vi "spindisk_unit_controller.vi"() -> ()   [LabVIEW 2016]
uses:
  <vilib>/Utility/error.llb/DialogType.ctl
  <vilib>/DAQmx/read.llb/DAQmx Read (Analog 1D DBL NChan 1Samp).vi
  <vilib>/DAQmx/miscellaneous.llb/DAQmx Fill In Error Info.vi
panel:
  in  "quit":bool
  in  "Spinning disk tab":enum32{"BD-CRVII", "ASI & Config File Info"}(tab)
  out "Ext Control Status":bool
  in  "Ext. analog control switch":bool
  in  "Analog control device":tag
  in  "Emission Filter":u16(ring) items=["Unknown Filter 1", "Unknown Filter 2", "Unknown Filter 3", "Unknown Filter 4", "Unknown Filter 5", "Unknown Filter 6", "Unknown Filter 7", "Unknown Filter 8"]
  in  "Dichroic Mirror":u16(ring) items=["Unknown Filter 1", "Unknown Filter 2", "Unknown Filter 3", "Unknown Filter 4", "Unknown Filter 5"]
  in  "Excitation Filter":u16(ring) items=["Unknown Filter 1", "Unknown Filter 2", "Unknown Filter 3", "Unknown Filter 4", "Unknown Filter 5", "Unknown Filter 6", "Unknown Filter 7", "Unknown Filter 8"]
  out "COM status":bool
  in  "Port Name":refnum<visa-resource-name>
  in  "Disk position":bool
  in  "Disk spinning":bool
  in  "Shutter":bool
  in  "init":bool
  in  "Ext. TTL Shutter\n Control":bool
  in  "ext. control update time (ms)":i32=50
  in  "serial response delay (ms)":u32
  in  "ext. cmd update delay (ms)":u32=500 max=1000
  out "cmd string":string
  out "Firmware Version":string
  out "query response":string
  out "ext. sig.\ncommitted":bool
  out "analog inputs":dbl[](array[numeric]) caption="analog \ninputs" format="%#1.3f"
  out "ASI REEPONSE":string
  out "ASI CMD":string
  in  "ASI Stage Port":refnum<visa-resource-name>
  in  "Set Backlash Values":bool
  in  "X backlash (um)":dbl min=0.0 max=200.0 step=0.5
  in  "Y backlash (um)":dbl min=0.0 max=200.0 step=0.5
  in  "Z backlash (um)":dbl=-40.0 min=-200.0 max=200.0 step=0.5
  out "Configuration file":string
  out "error out":errorcluster
  # "Programmed by Quan Qing\nQingLAB@ASU\nhttp://qinglab.physics.asu.edu\nquan.qing@asu.edu"
  # "ExFilter"
  # "EmFilter"
  # "DiMirror"
  # "DiskPos"
  # "DiskSpin"
  # "ASI backslash setting"
  # "Config. file information"
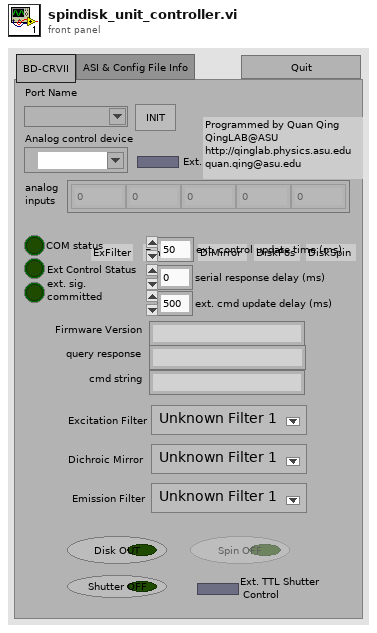
[diagram p1: front panel]
types:
  T1 = enum8{"Enabled", "Disabled", "Disabled and Grayed Out"}
  T2 = typedef "DialogType.ctl" = u16
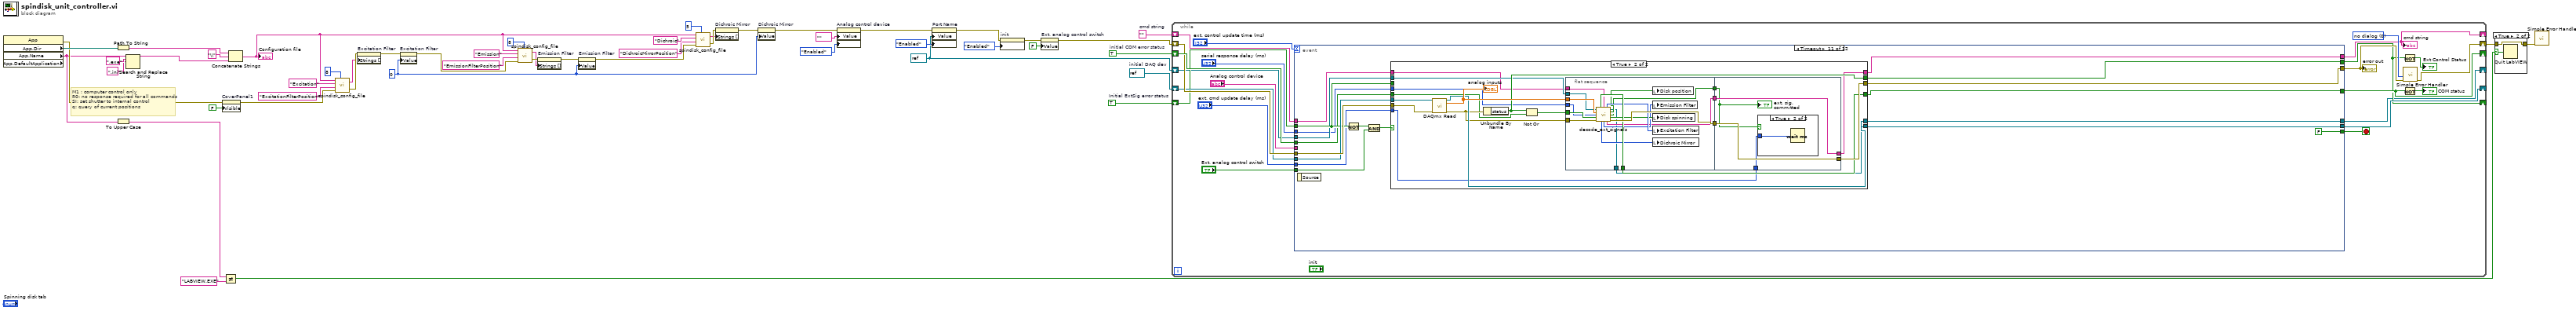
[diagram p0: block diagram]
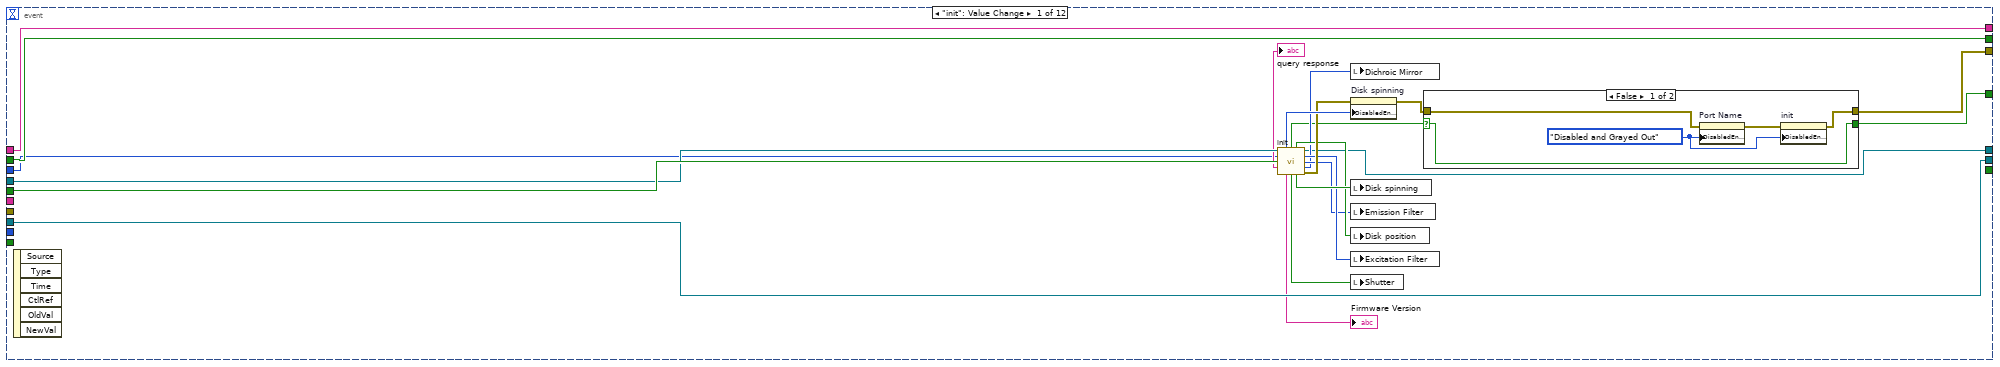
[diagram p3: hidden frame]
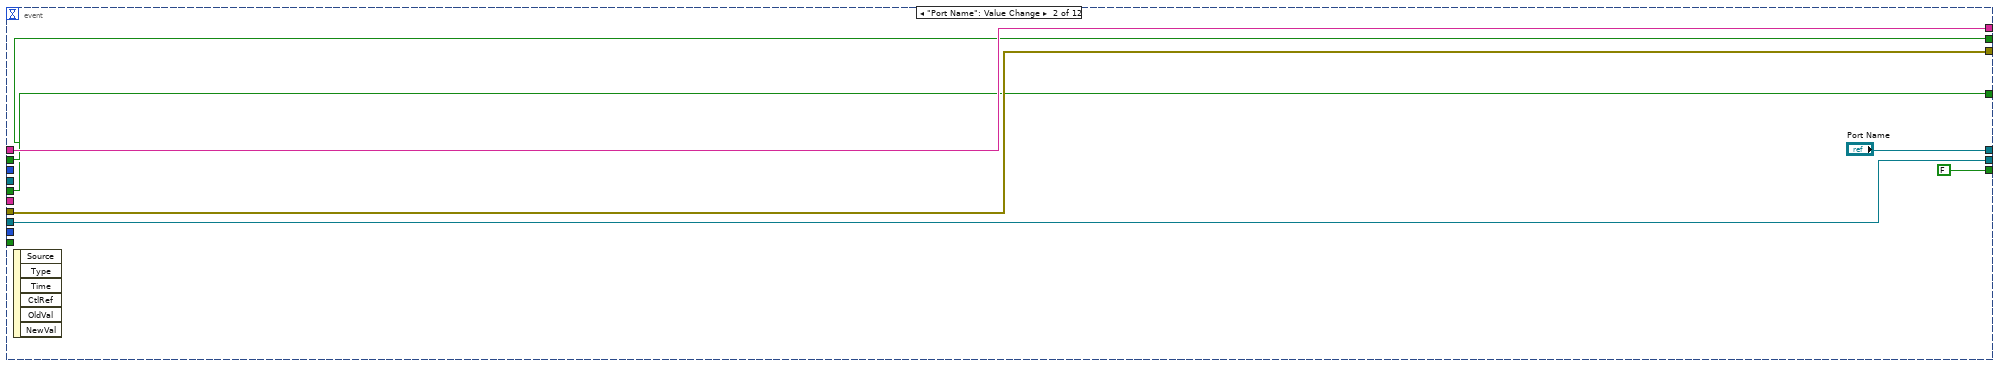
[diagram p5: hidden frame]
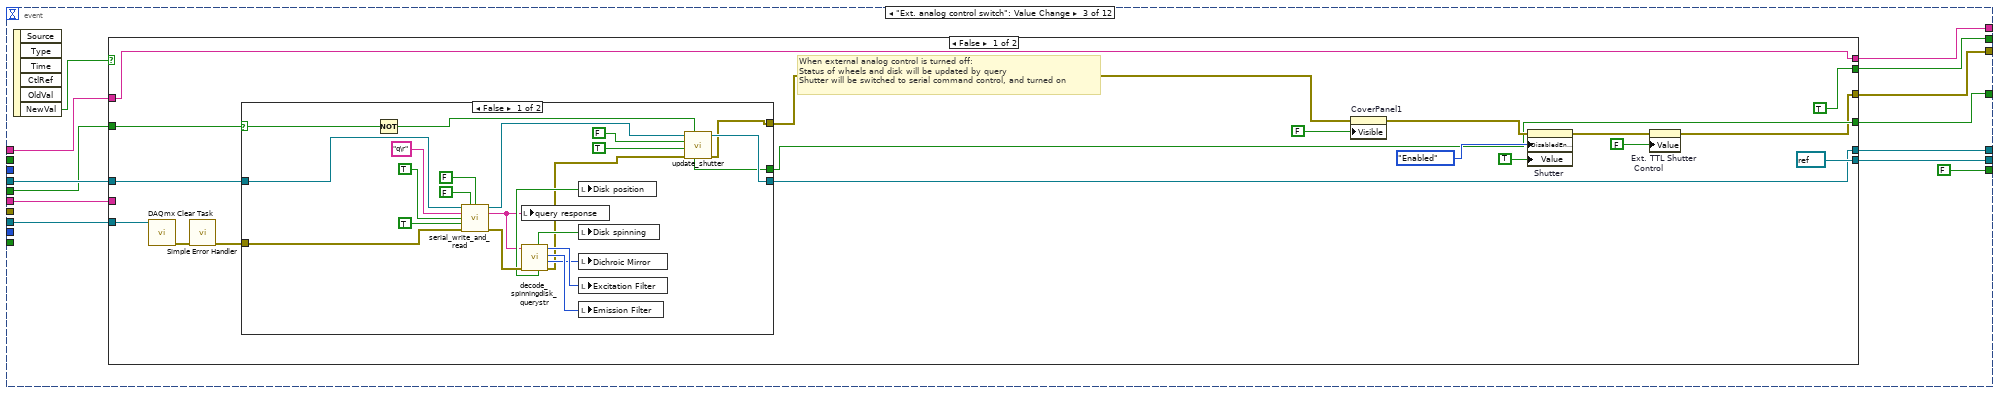
[diagram p6: hidden frame]
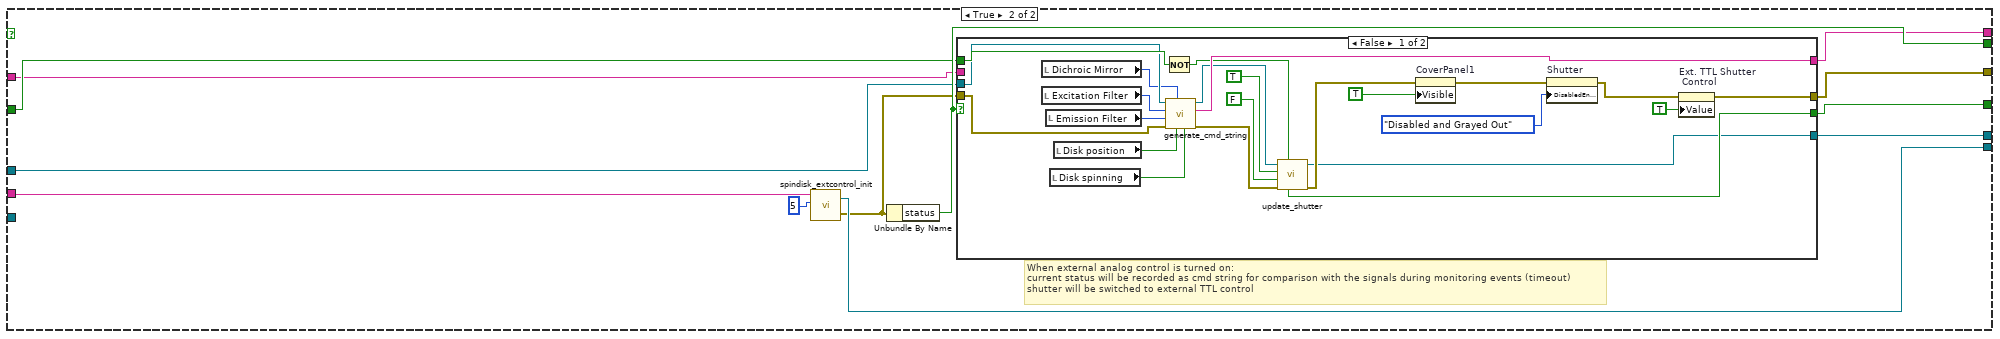
[diagram p8: hidden frame]
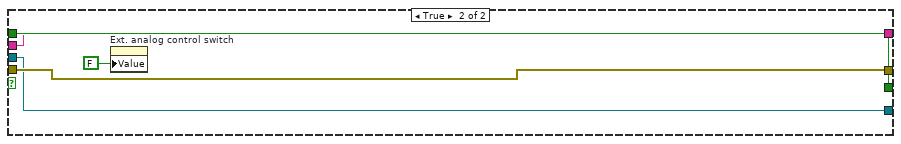
[diagram p9: hidden frame]
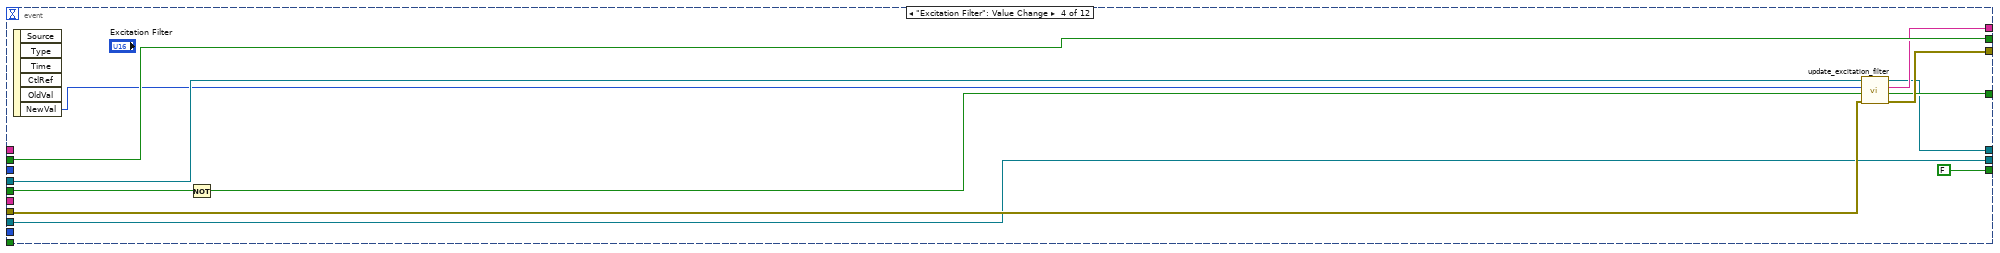
[diagram p10: hidden frame]
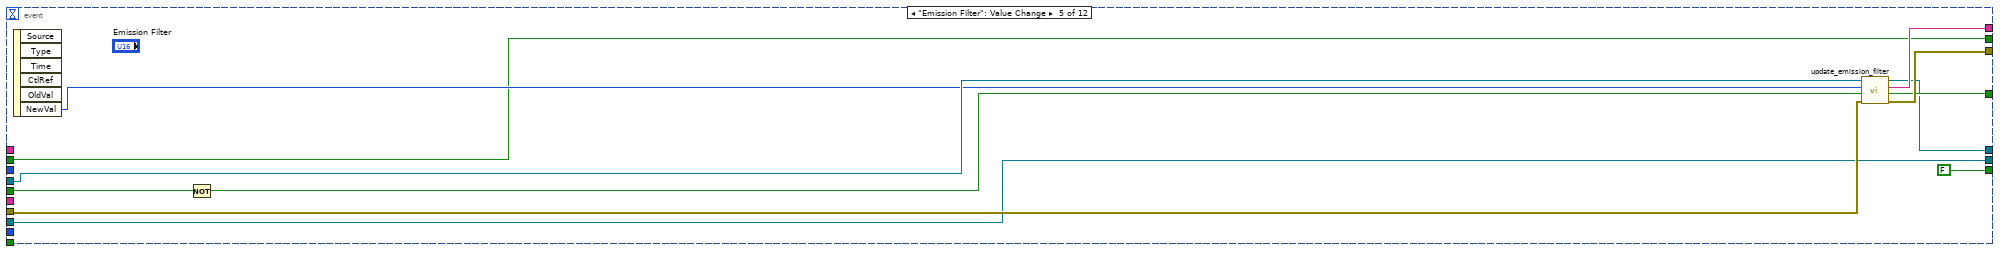
[diagram p11: hidden frame]
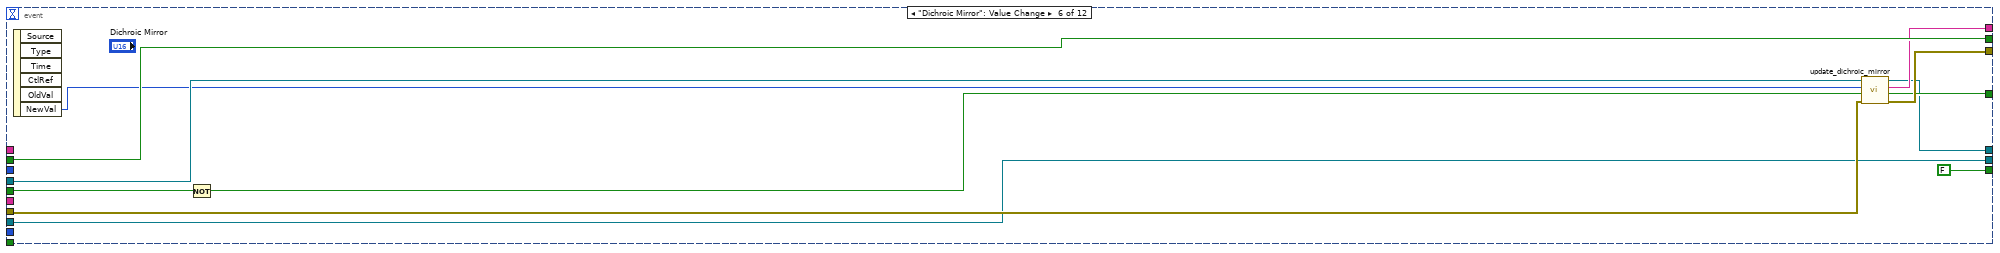
[diagram p12: hidden frame]
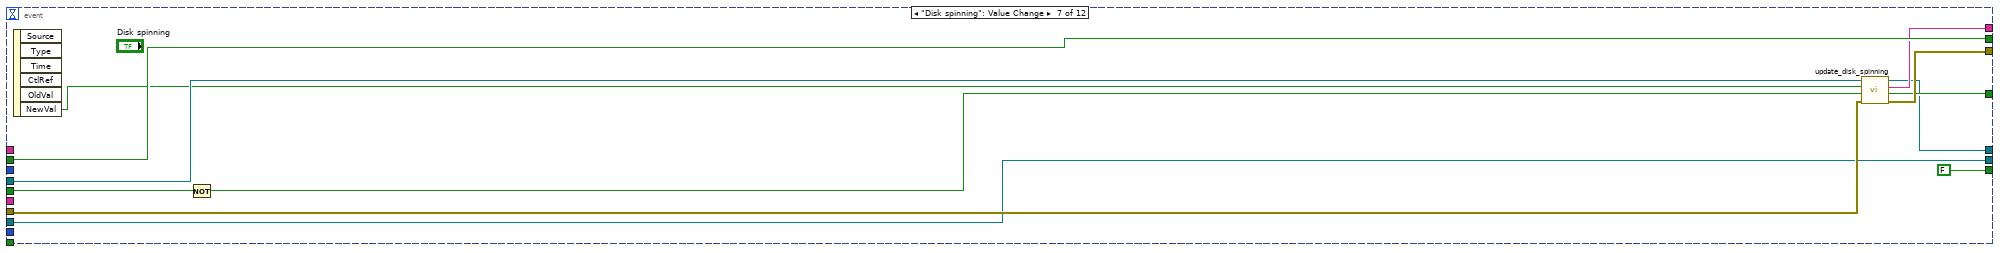
[diagram p13: hidden frame]
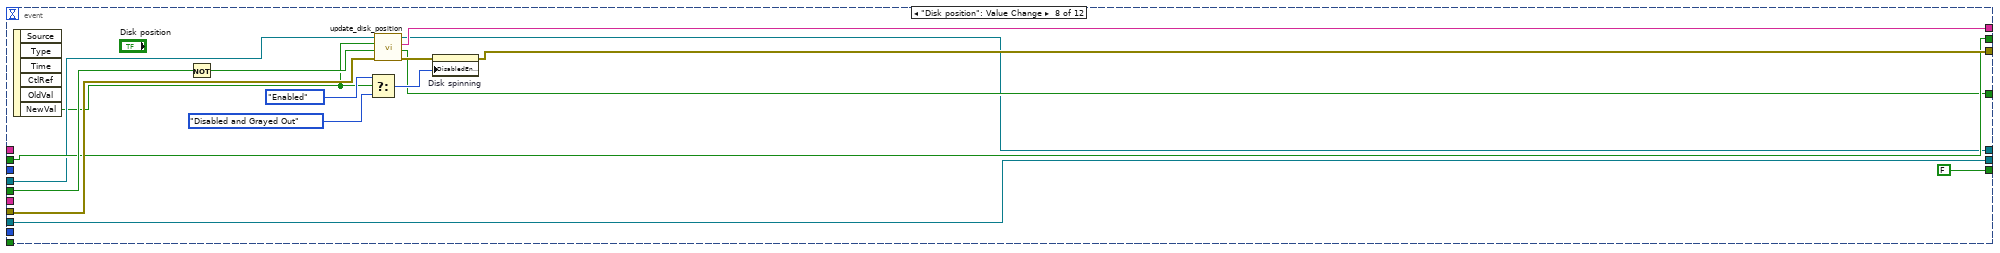
[diagram p14: hidden frame]
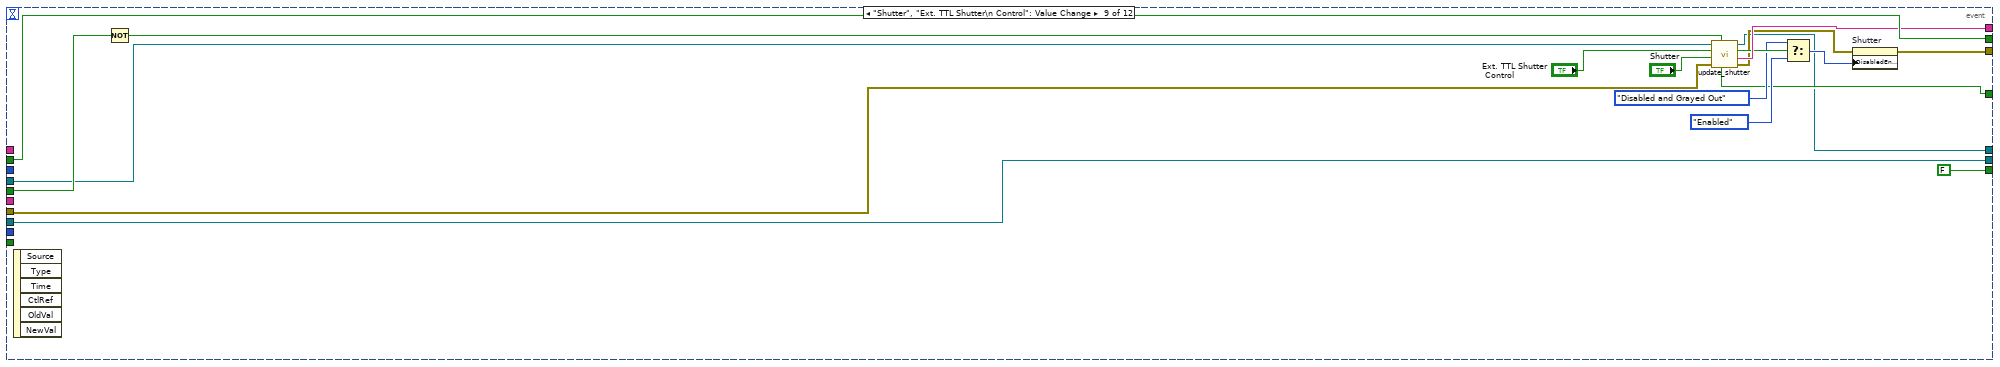
[diagram p15: hidden frame]
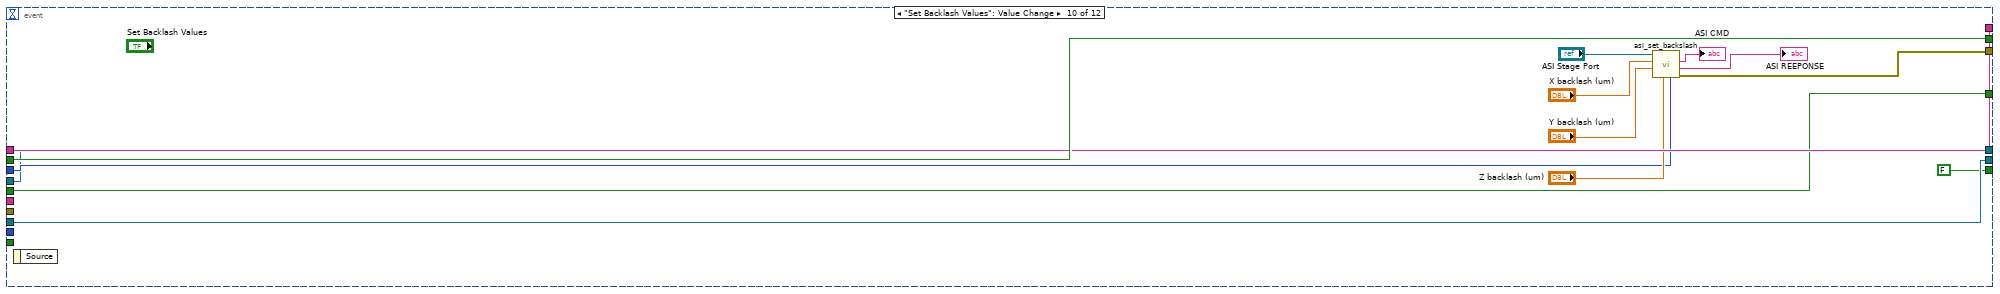
[diagram p16: hidden frame]
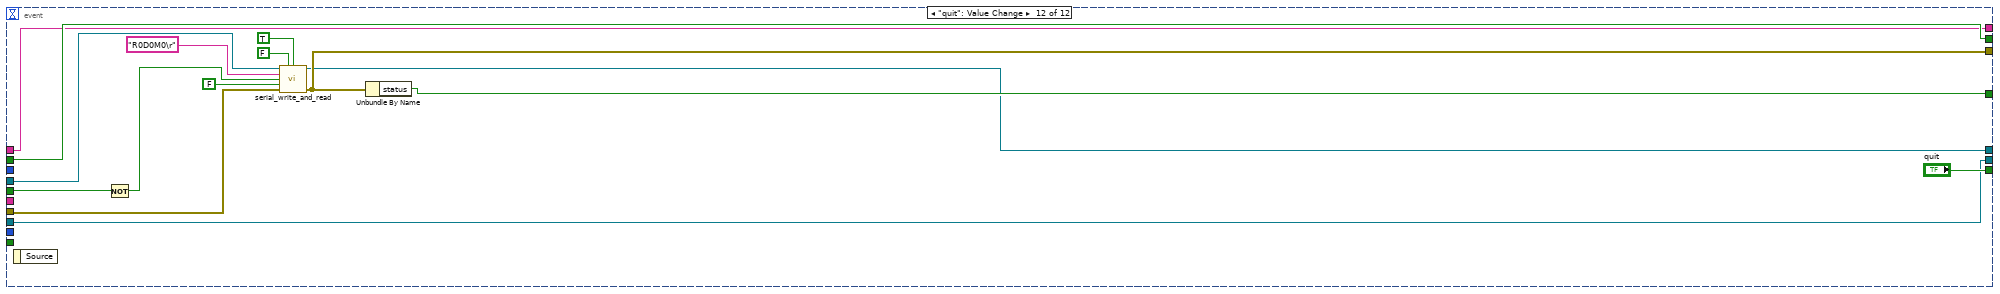
[diagram p19: hidden frame]
diagram:
  w3 = refnum<visa-resource-name> refnum ("Port Name")
  w16 = ""  # cmd string
  w19 = refnum<k21> refnum  # initial DAQ dev
  w18 = TRUE  # Initial ExtSig error status
  w26 = u16 0
  w36 = TRUE  # initial COM error status
  # "M1 : computer control only\nR0: no response required for all commands\nSI: set shutter to internal control\nq: query of current positions"
  n1 = property class="App" props=["App.Dir", "App.Name", "App.DefaultApplication"]() -> (error out=w15:errorcluster, "App.Dir"=w50:path, "App.Name"=w1:string)  [unwired: 2 in, 2 out]
  n2 = Path To String(path=w50) -> (string=w49:string)
  n3 = To Upper Case(1:w1) -> (0:w21:string)
  n4 = Search and Replace String(input string=w1, search string=".exe", replace string=".ini" ("replace string (\"\")")) -> (result string=w47:string)  [unwired: 5 in, 3 out]
  n5 = property on="CoverPanel1" class="SubPnl"(error in=w15, "Visible"=FALSE) -> (error out=w2:errorcluster)  [unwired: 1 in, 1 out]
  n6 = Not Equal?(x=w21, y="LABVIEW.EXE") -> (x != y?=w17:bool)
  n7 = Concatenate Strings(w49, "\\" ("string"), w47) -> (w42:string)
  "Configuration file" <- w42
  n8 = call "spindisk_config_file.vi"("config file path name"=w42, "section"="Excitation", "common_keyname"="ExcitationFilterPosition", "error in (no error)"=w2, "Positions"=8) -> ("filter list"=w25:string[], "error out"=w33:errorcluster)
  n9 = property on="Excitation Filter" class="Ring (strict)"(error in=w33, "Strings []"=w25) -> (error out=w34:errorcluster)  [unwired: 1 in, 1 out]
  n10 = property on="Excitation Filter" class="Ring (strict)"(error in=w34, "Value"=w26) -> (error out=w32:errorcluster)  [unwired: 1 in, 1 out]
  n11 = call "spindisk_config_file.vi"("config file path name"=w42, "section"="Emission", "common_keyname"="EmissionFilterPosition", "error in (no error)"=w32, "Positions"=8) -> ("filter list"=w24:string[], "error out"=w31:errorcluster)
  n12 = property on="Emission Filter" class="Ring (strict)"(error in=w31, "Strings []"=w24) -> (error out=w30:errorcluster)  [unwired: 1 in, 1 out]
  n13 = property on="Emission Filter" class="Ring (strict)"(error in=w30, "Value"=w26) -> (error out=w29:errorcluster)  [unwired: 1 in, 1 out]
  n14 = call "spindisk_config_file.vi"("config file path name"=w42, "section"="Dichroic", "common_keyname"="DichroicMirrorPosition", "error in (no error)"=w29, "Positions"=5) -> ("filter list"=w23:string[], "error out"=w28:errorcluster)
  n15 = property on="Dichroic Mirror" class="Ring (strict)"(error in=w28, "Strings []"=w23) -> (error out=w27:errorcluster)  [unwired: 1 in, 1 out]
  n16 = property on="Dichroic Mirror" class="Ring (strict)"(error in=w27, "Value"=w26) -> (error out=w7:errorcluster)  [unwired: 1 in, 1 out]
  n17 = property on="Analog control device" class="DAQmxName"(error in=w7, "Value"=tag "" ("Ext I/O device"), "DisabledEnum"=T1."Enabled" ("Disabled")) -> (error out=w6:errorcluster)  [unwired: 1 in, 1 out]
  n18 = property on="Port Name" class="VISAName"(error in=w6, "Value"=w3, "DisabledEnum"=T1."Enabled" ("Disabled")) -> (error out=w5:errorcluster)  [unwired: 1 in, 1 out]
  n19 = property on="init" class="Bool"(error in=w5, "DisabledEnum"=T1."Enabled" ("Disabled")) -> (error out=w4:errorcluster)  [unwired: 1 in, 1 out]
  n20 = property on="Ext. analog control switch" class="Bool (strict)"(error in=w4, "Value"=FALSE ("Ext. control enabled")) -> (error out=w13:errorcluster)  [unwired: 1 in, 1 out]
  n21 = while {
    shift-right: [w71] -> _
    shift-left: w36 -> [w73]
    shift-right: [w64] -> w22
    shift-left: w13 -> [w72]
    shift-right: [w68] -> _
    shift-left: w19 -> [w69]
    shift-right: [w62] -> _
    shift-left: w18 -> [w66]
    shift-right: [w59] -> _
    shift-left: w16 -> [w58]
    shift-right: [w53] -> _
    shift-left: w3 -> [w54]
    stop <- w74 stop-if-true
    w63 = T2 0 items=["no dialog", "OK message", "continue or stop message", "OK message + warnings", "continue/stop + warnings"] ("type of dialog (OK msg:1)")
    n22 = event shown="[10] Timeout" {
      selector: _ -> [_ _ _ _ _ _ _ _ _ _ _ _]
      dyn-events: _ -> [_ _ _ _ _ _ _ _ _ _ _ _]
      timeout: "ext. control update time (ms)" -> [_ _ _ _ _ _ _ _ _ _ _ _]
      tunnel: [_ FALSE ("quit") FALSE ("quit") FALSE ("quit") FALSE ("quit") FALSE ("quit") FALSE ("quit") FALSE ("quit") FALSE ("quit") FALSE ("quit") FALSE ("quit") "quit"] -> w74
      tunnel: [w78 w103 w114 w210 w222 w234 w246 w258 w275 w290 w312 w372] -> w71
      tunnel: w73 -> [w95 w103 w115 w214 w228 w240 w251 w268 w280 w290 w313 w375]
      tunnel: [w77 w108 w120 w218 w230 w242 w254 w269 w288 w302 w319 w373] -> w65
      tunnel: w72 -> [_ w108 _ w217 w229 w239 w252 w270 w287 _ w320 w381]
      tunnel: w69 -> [w94 w106 w122 w209 w220 w231 w245 w256 w272 w301 w318 w367]
      tunnel: [w94 w106 w121 w209 w220 w231 w245 w256 w272 w301 w317 w367] -> w68
      tunnel: [w91 w104 w119 w216 w223 w241 w253 w267 w286 w300 w311 w380] -> w62
      tunnel: w66 -> [w91 w104 _ w216 w223 w241 w253 w267 w286 w300 w314 w380]
      tunnel: w54 -> [w90 _ w116 w212 w225 w236 w248 w260 w278 w289 w310 w369]
      tunnel: "Analog control device" -> [_ _ w118 _ _ _ _ _ _ _ _ _]
      tunnel: "Ext. analog control switch" -> [_ _ _ _ _ _ _ _ _ _ w309 _]
      tunnel: [w81 w107 w112 w215 w227 w238 w250 w266 w285 w297 w308 w370] -> w59
      tunnel: w58 -> [w81 w107 w113 _ _ _ _ _ _ w297 w307 w370]
      tunnel: "ext. cmd update delay (ms)" -> [_ _ _ _ _ _ _ _ _ _ w306 _]
      tunnel: "serial response delay (ms)" -> [w76 _ _ _ _ _ _ _ _ w292 w305 _]
      tunnel: [w75 "Port Name" w111 w208 w221 w232 w244 w257 w273 w289 w303 w368] -> w53
      event "init": Value Change {
        n23 = event-data() -> ()  [unwired: 1 in, 6 out]
        n24 = call "init.vi"("Port Name"=w90, "COM response delay"=w76, "current error status"=w95) -> ("disk spinning disable state"=w93:T1, "new error status"=w80:bool, "Disk position"=w87:bool, "VISA resource name out"=w75:refnum<visa-resource-name>, "Excitation Filter"=w86:u16, "Emission Filter"=w85:u16, "query response"=→"query response":string, "Dichroic Mirror"=w84:u16, "Firmware Version"=→"Firmware Version":string, "Shutter"=w89:bool, "Disk spinning"=w88:bool, "error out"=w92:errorcluster)  [unwired: 1 in]
        n25 = local write "Dichroic Mirror"(w84) -> ()
        n26 = property on="Disk spinning" class="Bool (strict)"(error in=w92, "DisabledEnum"=w93) -> (error out=w79:errorcluster)  [unwired: 1 in, 1 out]
        n27 = local write "Disk spinning"(w88) -> ()
        n28 = local write "Emission Filter"(w85) -> ()
        n29 = local write "Disk position"(w87) -> ()
        n30 = local write "Excitation Filter"(w86) -> ()
        n31 = local write "Shutter"(w89) -> ()
        n32 = case shown="False" w80 {
          selector: w80 -> [w100 w102]
          tunnel: w79 -> [w99 w101]
          tunnel: [w100 w102] -> w78
          tunnel: [w97 w101] -> w77
          frame False {
            w96 = T1."Disabled and Grayed Out" ("Disabled")
            n33 = property on="Port Name" class="VISAName"(error in=w99, "DisabledEnum"=w96) -> (error out=w98:errorcluster)  [unwired: 1 in, 1 out]
            n34 = property on="init" class="Bool"(error in=w98, "DisabledEnum"=w96) -> (error out=w97:errorcluster)  [unwired: 1 in, 1 out]
          }
          frame True {
          }
        }
      }
      event "Port Name": Value Change {
        n35 = event-data() -> ()  [unwired: 1 in, 6 out]
      }
      event "Ext. analog control switch": Value Change {
        n36 = event-data() -> ("NewVal"=w117:bool)  [unwired: 1 in, 5 out]
        n37 = case shown="False" w117 {
          tunnel: w118 -> [_ w178]
          tunnel: [w125 w173] -> w120
          tunnel: [refnum<k21> refnum ("task out") w176] -> w121
          tunnel: w122 -> [w140 _]
          tunnel: [TRUE ("status") w175] -> w119
          tunnel: w116 -> [w127 w172]
          tunnel: w115 -> [w124 w171]
          tunnel: [w126 w170] -> w114
          tunnel: w113 -> [w130 w169]
          tunnel: [w130 w168] -> w112
          tunnel: [w123 w167] -> w111
          frame False {
            # "When external analog control is turned off:\nStatus of wheels and disk will be updated by query\nShutter will be switched to serial command control, and turned on"
            n38 = call <vilib>:"DAQmx Clear Task.vi"("task in"=w140) -> ("error out"=w139:errorcluster)  [unwired: 14 in]
            n39 = call <vilib>:"Simple Error Handler.vi"("error in (no error)"=w139) -> ("error out"=w129:errorcluster)  [unwired: 4 in, 4 out]
            n40 = case shown="False" w124 {
              selector: w124 -> [w146 w164]
              tunnel: w129 -> [w157 w165]
              tunnel: [w143 w165] -> w128
              tunnel: w127 -> [w156 w166]
              tunnel: [w147 w166] -> w123
              tunnel: [w145 w164] -> w126
              frame False {
                n41 = Not(x=w146) -> (.not. x?=w142:bool)
                n42 = call "serial_write_and_read.vi"("port name in"=w156, "reconnect?"=FALSE, "disconnect?"=FALSE, "write buffer"="q\r", "do writing?"=TRUE, "expecting response?"=TRUE, "error in"=w157) -> ("port name out"=w148:refnum<visa-resource-name>, "read buffer"=w141:string, "error out"=w159:errorcluster)  [unwired: 6 in]
                n43 = local write "query response"(w141) -> ()
                n44 = call "decode_spinningdisk_querystr.vi"("input string"=w141, "error in"=w159) -> ("disk spinning"=w151:bool, "disk position"=w152:bool, "excitation filter"=w154:u16, "emission filter"=w155:u16, "dichroic mirror"=w153:u16, "error out"=w144:errorcluster)  [unwired: 2 in, 1 out]
                n45 = local write "Disk position"(w152) -> ()
                n46 = local write "Disk spinning"(w151) -> ()
                n47 = local write "Dichroic Mirror"(w153) -> ()
                n48 = local write "Excitation Filter"(w154) -> ()
                n49 = local write "Emission Filter"(w155) -> ()
                n50 = call "update_shutter.vi"("commit?"=w142, "error in"=w144, "Shutter"=TRUE, "TTL external control?"=FALSE, "port in"=w148) -> ("error out"=w143:errorcluster, "port out"=w147:refnum<visa-resource-name>, "update COM error status"=w145:bool)  [unwired: 2 out]
              }
              frame True {
              }
            }
            n51 = property on="CoverPanel1" class="SubPnl"(error in=w128, "Visible"=FALSE) -> (error out=w132:errorcluster)  [unwired: 1 in, 1 out]
            n52 = property on="Shutter" class="Bool (strict)"(error in=w132, "DisabledEnum"=T1."Enabled" ("Disabled"), "Value"=TRUE ("Shutter")) -> (error out=w136:errorcluster)  [unwired: 1 in, 1 out]
            n53 = property on="Ext. TTL Shutter\n Control" class="Bool (strict)"(error in=w136, "Value"=FALSE ("TTL Shutter Control")) -> (error out=w125:errorcluster)  [unwired: 1 in, 1 out]
          }
          frame True {
            # "When external analog control is turned on:\ncurrent status will be recorded as cmd string for comparison with the signals during monitoring events (timeout)\nshutter will be switched to external TTL control"
            n54 = call "spindisk_extcontrol_init.vi"("Choose Device"=w178, "Analog input number"=5) -> ("task out"=w176:refnum<k21>, "error out"=w174:errorcluster)  [unwired: 3 in]
            n55 = Unbundle By Name(w174) -> ("status"=w175:bool)
            n56 = case shown="False" w175 {
              tunnel: w174 -> [w195 w204]
              tunnel: [w187 w204] -> w173
              tunnel: w172 -> [w194 w202]
              tunnel: w171 -> [w199 w206]
              tunnel: [w181 w206] -> w170
              tunnel: w169 -> [_ w203]
              tunnel: [w193 w203] -> w168
              tunnel: [w179 w202] -> w167
              frame False {
                n57 = local read "Dichroic Mirror"() -> (w192:u16)
                n58 = local read "Excitation Filter"() -> (w190:u16)
                n59 = local read "Emission Filter"() -> (w189:u16)
                n60 = local read "Disk spinning"() -> (w191:bool)
                n61 = local read "Disk position"() -> (w188:bool)
                n62 = Not(x=w199) -> (.not. x?=w180:bool)
                n63 = call "generate_cmd_string.vi"("disk spinning"=w191, "disk position"=w188, "dichroic mirror"=w192, "error in (no error)"=w195, "emission filter"=w189, "excitation filter"=w190, "port in"=w194) -> ("error out"=w183:errorcluster, "cmd string"=w193:string, "port out"=w184:refnum<visa-resource-name>)  [unwired: 2 in]
                n64 = call "update_shutter.vi"("commit?"=w180, "error in"=w183, "Shutter"=FALSE, "TTL external control?"=TRUE, "port in"=w184) -> ("error out"=w182:errorcluster, "port out"=w179:refnum<visa-resource-name>, "update COM error status"=w181:bool)  [unwired: 2 out]
                n65 = property on="CoverPanel1" class="SubPnl"(error in=w182, "Visible"=TRUE) -> (error out=w197:errorcluster)  [unwired: 1 in, 1 out]
                n66 = property on="Shutter" class="Bool (strict)"(error in=w197, "DisabledEnum"=T1."Disabled and Grayed Out" ("Disabled")) -> (error out=w201:errorcluster)  [unwired: 1 in, 1 out]
                n67 = property on="Ext. TTL Shutter\n Control" class="Bool (strict)"(error in=w201, "Value"=TRUE ("TTL Shutter Control")) -> (error out=w187:errorcluster)  [unwired: 1 in, 1 out]
              }
              frame True {
                n68 = property on="Ext. analog control switch" class="Bool (strict)"("Value"=FALSE ("Ext. control enabled")) -> ()  [unwired: 2 in, 2 out]
              }
            }
          }
        }
      }
      event "Excitation Filter": Value Change {
        n69 = event-data() -> ("NewVal"=w211:u16)  [unwired: 1 in, 5 out]
        n70 = Not(x=w214) -> (.not. x?=w213:bool)
        n71 = call "update_excitation_filter.vi"("error in (no error)"=w217, "commit?"=w213, "excitation filter #"=w211, "VISA resource name"=w212) -> ("error out"=w218:errorcluster, "update COM error status"=w210:bool, "cmd string"=w215:string, "VISA resource name out"=w208:refnum<visa-resource-name>)
      }
      event "Emission Filter": Value Change {
        n72 = event-data() -> ("NewVal"=w224:u16)  [unwired: 1 in, 5 out]
        n73 = Not(x=w228) -> (.not. x?=w226:bool)
        n74 = call "update_emission_filter.vi"("error in (no error)"=w229, "commit?"=w226, "emission filter #"=w224, "VISA resource name"=w225) -> ("error out"=w230:errorcluster, "update COM error status"=w222:bool, "cmd string"=w227:string, "VISA resource name out"=w221:refnum<visa-resource-name>)
      }
      event "Dichroic Mirror": Value Change {
        n75 = event-data() -> ("NewVal"=w235:u16)  [unwired: 1 in, 5 out]
        n76 = Not(x=w240) -> (.not. x?=w237:bool)
        n77 = call "update_dichroic_mirror.vi"("error in (no error)"=w239, "commit?"=w237, "dichroic mirror #"=w235, "VISA resource name"=w236) -> ("error out"=w242:errorcluster, "update COM error status"=w234:bool, "cmd string"=w238:string, "VISA resource name out"=w232:refnum<visa-resource-name>)
      }
      event "Disk spinning": Value Change {
        n78 = event-data() -> ("NewVal"=w247:bool)  [unwired: 1 in, 5 out]
        n79 = Not(x=w251) -> (.not. x?=w249:bool)
        n80 = call "update_disk_spinning.vi"("error in (no error)"=w252, "commit?"=w249, "disk spinning"=w247, "VISA resource name"=w248) -> ("error out"=w254:errorcluster, "update COM error status"=w246:bool, "cmd string"=w250:string, "VISA resource name out"=w244:refnum<visa-resource-name>)
      }
      event "Disk position": Value Change {
        n81 = event-data() -> ("NewVal"=w259:bool)  [unwired: 1 in, 5 out]
        n82 = Not(x=w268) -> (.not. x?=w265:bool)
        n83 = Select(t=T1."Enabled" ("Disabled"), s=w259, f=T1."Disabled and Grayed Out" ("Disabled")) -> (s? t:f=w264:T1)
        n84 = call "update_disk_position.vi"("error in (no error)"=w270, "commit?"=w265, "disk position"=w259, "VISA resource name"=w260) -> ("error out"=w263:errorcluster, "update COM error status"=w258:bool, "cmd string"=w266:string, "VISA resource name out"=w257:refnum<visa-resource-name>)
        n85 = property on="Disk spinning" class="Bool (strict)"(error in=w263, "DisabledEnum"=w264) -> (error out=w269:errorcluster)  [unwired: 1 in, 1 out]
      }
      event "Shutter", "Ext. TTL Shutter\n Control": Value Change {
        n86 = event-data() -> ()  [unwired: 1 in, 6 out]
        n87 = Not(x=w280) -> (.not. x?=w274:bool)
        n88 = call "update_shutter.vi"("commit?"=w274, "error in"=w287, "Shutter"="Shutter", "TTL external control?"="Ext. TTL Shutter\n Control", "port in"=w278) -> ("error out"=w279:errorcluster, "cmd string"=w285:string, "disable shutter button?"=w284:bool, "port out"=w273:refnum<visa-resource-name>, "update COM error status"=w275:bool)
        n89 = Select(t=T1."Disabled and Grayed Out" ("Disabled"), s=w284, f=T1."Enabled" ("Disabled")) -> (s? t:f=w281:T1)
        n90 = property on="Shutter" class="Bool (strict)"(error in=w279, "DisabledEnum"=w281) -> (error out=w288:errorcluster)  [unwired: 1 in, 1 out]
      }
      event "Set Backlash Values": Value Change {
        n91 = event-data() -> ()  [unwired: 1 in, 1 out]
        n92 = call "asi_set_backslash.vi"("COM response delay"=w292, "Z backlash (um)"="Z backlash (um)", "Y backlash (um)"="Y backlash (um)", "X backlash (um)"="X backlash (um)", "ASI Stage Port"="ASI Stage Port") -> ("error out"=w302:errorcluster, "RESPONSE"=→"ASI REEPONSE":string, "CMD"=→"ASI CMD":string)  [unwired: 4 in]
      }
      event Timeout {
        n93 = event-data() -> ()  [unwired: 1 in, 1 out]
        n94 = Not(x=w314) -> (.not. x?=w315:bool)
        n95 = And(x=w315, y=w309) -> (x .and. y?=w316:bool)
        n96 = case shown="True" w316 {
          tunnel: w320 -> [w326 w341]
          tunnel: [w326 w344] -> w319
          tunnel: [w323 w335] -> w312
          tunnel: w318 -> [w325 w345]
          tunnel: [w325 w342] -> w317
          tunnel: w314 -> [w324 _]
          tunnel: w313 -> [w323 w339]
          tunnel: [w324 w338] -> w311
          tunnel: w310 -> [w321 w337]
          tunnel: [w322 w334] -> w308
          tunnel: w307 -> [w322 w330]
          tunnel: w306 -> [_ w331]
          tunnel: w305 -> [_ w328]
          tunnel: [w321 w327] -> w303
          frame False {
          }
          frame True {
            n97 = call-poly <vilib>:"DAQmx Read.vi"("task/channels in"=w345, "error in"=w341) -> ("task out"=w342:refnum<k21>, "data"=w343:dbl[], "error out"=w340:errorcluster)  [unwired: 11 in]
            "analog inputs" <- w343
            n98 = Unbundle By Name(w340) -> ("status"=w338:bool)
            n99 = Not Or(1:w339, 2:w338) -> (0:w336:bool)
            n100 = flat-sequence {
              tunnel: w343 -> [w360]
              tunnel: w340 -> [w359]
              tunnel: w337 -> [w358]
              tunnel: w336 -> [w357]
              tunnel: [w356] -> w335
              tunnel: [w361] -> w333
              tunnel: [w350] -> w332
              tunnel: w330 -> [w349]
              tunnel: [w348] -> w329
              tunnel: w328 -> [w347]
              tunnel: [w346] -> w327
              tunnel: [w364] -> w334
              tunnel: [w365] -> w344
              tunnel: w333 -> [w365]
              tunnel: w332 -> [w364]
              tunnel: w331 -> [w363]
              tunnel: w329 -> [w362]
              frame #0 {
                n101 = call "decode_ext_signals.vi"("VISA resource name"=w358, "previous_status cmd string"=w349, "analog inputs"=w360, "COM response delay"=w347, "commit?"=w357, "error in (no error)"=w359) -> ("update of COM error status"=w356:bool, "excitation filter"=w355:u16, "VISA resource name out"=w346:refnum<visa-resource-name>, "disk position"=w354:bool, "update need commit?"=w348:bool, "disk spinning"=w353:bool, "dichroic mirror"=w352:u16, "emission filter"=w351:u16, "cmd string"=w350:string, "error out"=w361:errorcluster)
                n102 = local write "Disk position"(w354) -> ()
                n103 = local write "Emission Filter"(w351) -> ()
                n104 = local write "Disk spinning"(w353) -> ()
                n105 = local write "Excitation Filter"(w355) -> ()
                n106 = local write "Dichroic Mirror"(w352) -> ()
              }
              frame #1 {
                n107 = case shown="True" w362 {
                  tunnel: w363 -> [_ w366]
                  frame False {
                  }
                  frame True {
                    n108 = Wait (ms)(milliseconds to wait=w366) -> ()  [unwired: 1 out]
                  }
                }
                "ext. sig.\ncommitted" <- w362
              }
            }
          }
        }
      }
      event "quit": Value Change {
        n109 = event-data() -> ()  [unwired: 1 in, 1 out]
        n110 = Not(x=w375) -> (.not. x?=w374:bool)
        n111 = call "serial_write_and_read.vi"("port name in"=w369, "reconnect?"=FALSE, "disconnect?"=TRUE, "write buffer"="R0D0M0\r", "do writing?"=w374, "expecting response?"=FALSE, "error in"=w381) -> ("port name out"=w368:refnum<visa-resource-name>, "error out"=w373:errorcluster)  [unwired: 6 in, 1 out]
        n112 = Unbundle By Name(w373) -> ("status"=w372:bool)
      }
    }
    "error out" <- w65
    "cmd string" <- w59
    n113 = Not(x=w62) -> (.not. x?=→"Ext Control Status":bool)
    n114 = Not(x=w71) -> (.not. x?=→"COM status":bool)
    n115 = call <vilib>:"Simple Error Handler.vi"("type of dialog (OK msg:1)"=w63, "error in (no error)"=w65) -> ("error out"=w64:errorcluster)  [unwired: 3 in, 4 out]
  }
  n116 = case shown="True" w17 {
    selector: w17 -> [_ w384]
    tunnel: w22 -> [w382 w383]
    tunnel: [w382 w383] -> w35
    frame False {
    }
    frame True {
      n117 = Quit LabVIEW(quit? (T)=w384) -> ()
    }
  }
  n118 = call <vilib>:"Simple Error Handler.vi"("error in (no error)"=w35) -> ()  [unwired: 4 in, 5 out]
